vi "read_4ch.vi"(10 "channel offsets":T1) -> (2 "read output":T1)   [LabVIEW 2010]
uses:
  common_typedefs/channels_cluster.ctl
  <vilib>/eio/EIONode/EIONode.xnode
  <vilib>/rvi/eio/nirviEIOImplementation/nirviEIOImplementation.xnode
  <vilib>/rvi/eio/common/nirviEmuClasses.ctl
  <vilib>/rvi/eio/common/nirviEmuTemplateMethod_noerrors.vi
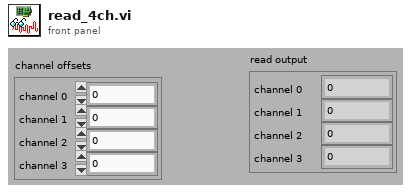
[diagram p1: front panel]
types:
  T1 = typedef "channels_cluster.ctl" = cluster{"channel 0":u32, "channel 1":u32, "channel 2":u32, "channel 3":u32}
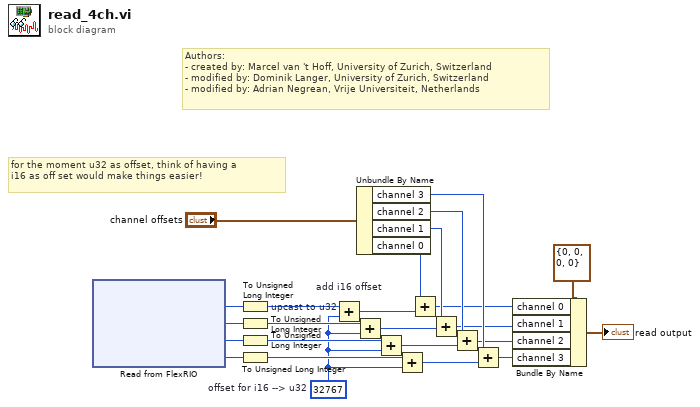
[diagram p0: block diagram]
diagram:
  w10 = u32 32767  # offset for i16 --> u32
  # "for the moment u32 as offset, think of having a\ni16 as off set would make things easier!"
  # "Authors: \n- created by: Marcel van 't Hoff, University of Zurich, Switzerland\n- modified by: Dominik Langer, University of Zurich, Switzerland\n- modified by: Adrian Negrean, Vrije Universiteit, Netherlands"
  n1 = xnode "Read from FlexRIO"() -> ("IO Module\\AI A0"=w14:i16, "IO Module\\AI A1"=w15:i16, "IO Module\\AI A2"=w16:i16, "IO Module\\AI A3"=w20:i16)  [unwired: 4 in, 4 out]
  n2 = To Unsigned Long Integer "upcast to u32"(number=w14) -> (unsigned 32bit integer=w13:u32)
  n3 = To Unsigned Long Integer(number=w15) -> (unsigned 32bit integer=w12:u32)
  n4 = To Unsigned Long Integer(number=w16) -> (unsigned 32bit integer=w11:u32)
  n5 = To Unsigned Long Integer(number=w20) -> (unsigned 32bit integer=w21:u32)
  n6 = Add "add i16 offset"(x=w13, y=w10) -> (x+y=w9:u32)
  n7 = Add(x=w12, y=w10) -> (x+y=w8:u32)
  n8 = Unbundle By Name("channel offsets") -> ("channel 3"=w19:u32, "channel 2"=w6:u32, "channel 1"=w5:u32, "channel 0"=w4:u32)
  n9 = Add(x=w11, y=w10) -> (x+y=w7:u32)
  n10 = Add(x=w21, y=w10) -> (x+y=w18:u32)
  n11 = Add(x=w4, y=w9) -> (x+y=w3:u32)
  n12 = Add(x=w5, y=w8) -> (x+y=w2:u32)
  n13 = Add(x=w6, y=w7) -> (x+y=w1:u32)
  n14 = Add(x=w19, y=w18) -> (x+y=w17:u32)
  n15 = Bundle By Name(cluster=T1 {"channel 0"=0, "channel 1"=0, "channel 2"=0, "channel 3"=0} ("read output"), "channel 0"=w3, "channel 1"=w2, "channel 2"=w1, "channel 3"=w17) -> (→"read output":T1)
